vi "conv-var_vers_POP.vi"(7 "Variable":string) -> (1 "Pop/Ech (Ch)":string, 2 "Pop ?":bool, 3 "pop/ech":T1)   [LabVIEW 2010, in "lv_04.lvlib"]
uses:
  lv_04.lvlib
  commandes/c_enum_pop-ech.ctl
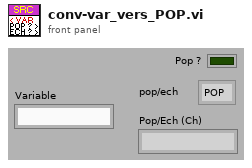
[diagram p1: front panel]
types:
  T1 = typedef "lv_04.lvlib/c_enum_pop-ech.ctl" = enum16{"POP", "ECH"}
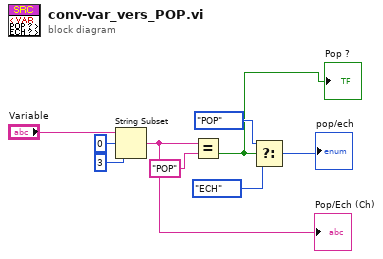
[diagram p0: block diagram]
diagram:
  n1 = String Subset(string="Variable", offset (0)=0, length (rest)=3 ("longueur (reste)")) -> (substring=w3:string)
  "Pop/Ech (Ch)" <- w3
  n2 = Equal?(x=w3, y="POP") -> (x = y?=w1:bool)
  "Pop ?" <- w1
  n3 = Select(t=c_enum_pop-ech."POP" ("pop/ech"), s=w1, f=c_enum_pop-ech."ECH" ("pop/ech")) -> (s? t:f=→"pop/ech":T1)
